vi "FRCts20_Backend_ClosedRequests.vi"(6 "Message Attributes":T1, 8 "error in (no error)":errorcluster, 10 "Data":string, 11 "Engine_Refnums":T2) -> (0 "error out":errorcluster)   [LabVIEW 2013, in "FRCts20_Backend_Engine.lvlib"]
uses:
  FRCts20_Backend_Engine.lvlib
  FRCts20_Backend_EngineRefnums.ctl
  INI_Accessor/FRCts20_Backend_INI Controller.lvclass
  Dependencies/AMC/_SubVIs/TypeDefs/Message Queue.ctl
  Dependencies/AMC/_SubVIs/TypeDefs/Message.ctl
  Dependencies/Keyed Array/KeyedArray.ctl
  <vilib>/addons/database/Connection.llb/Conn ObjectReference.ctl
  FRCts20_Backend_FGVOperation.ctl
  FRCts20_Backend_API/FRCts20_Backend_API_ClosedRequests.ctl
  FRCts20_Backend_API/FRCts20_Backend_API.lvlib
  Dependencies/Keyed Array/Tools_KeyedArray.lvlib
  Dependencies/AMC/AMC.lvlib
  <vilib>/addons/database/NI_Database_API.lvlib
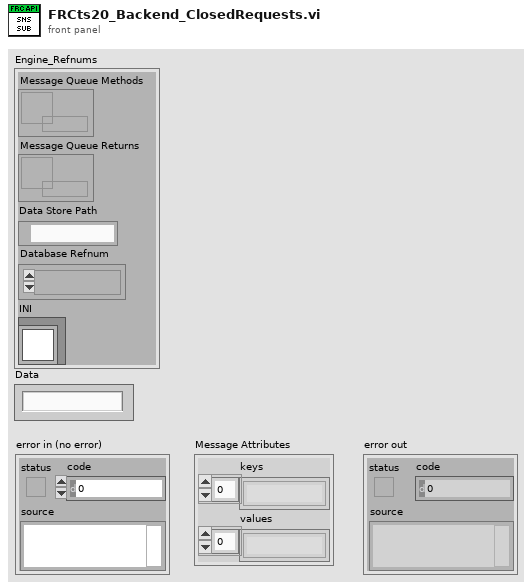
[diagram p1: front panel]
types:
  T1 = typedef "Tools_KeyedArray.lvlib/KeyedArray.ctl" = cluster{"keys":string[], "values":string[]}
  T2 = typedef "FRCts20_Backend_Engine.lvlib/FRCts20_Backend_EngineRefnums.ctl" = cluster{"Message Queue Methods":T3, "Message Queue Returns":T3, "Data Store Path":path, "Database Refnum":T4, "INI":refnum<class "FRCts20_Backend_INI Controller.lvclass">}
  T3 = typedef "AMC.lvlib/Message Queue.ctl" = refnum<queue>
  T4 = typedef "NI_Database_API.lvlib/Conn ObjectReference.ctl" = refnum<k1>
  T5 = typedef "FRCts20_Backend_API.lvlib/FRCts20_Backend_API_ClosedRequests.ctl" = cluster{"Event Name":string, "APIReturn":string, "Array of Requests":cluster{"Team Number":string, "ReqNumber":string, "Request":string, "OpenDate":string, "CloseDate":string}[]}
  T6 = typedef "FRCts20_Backend_Engine.lvlib/FRCts20_Backend_FGVOperation.ctl" = enum16{"Initialize", "EnqueueMessage", "EnqueueDataReturn", "FlushMessage", "FlushDataReturn"}
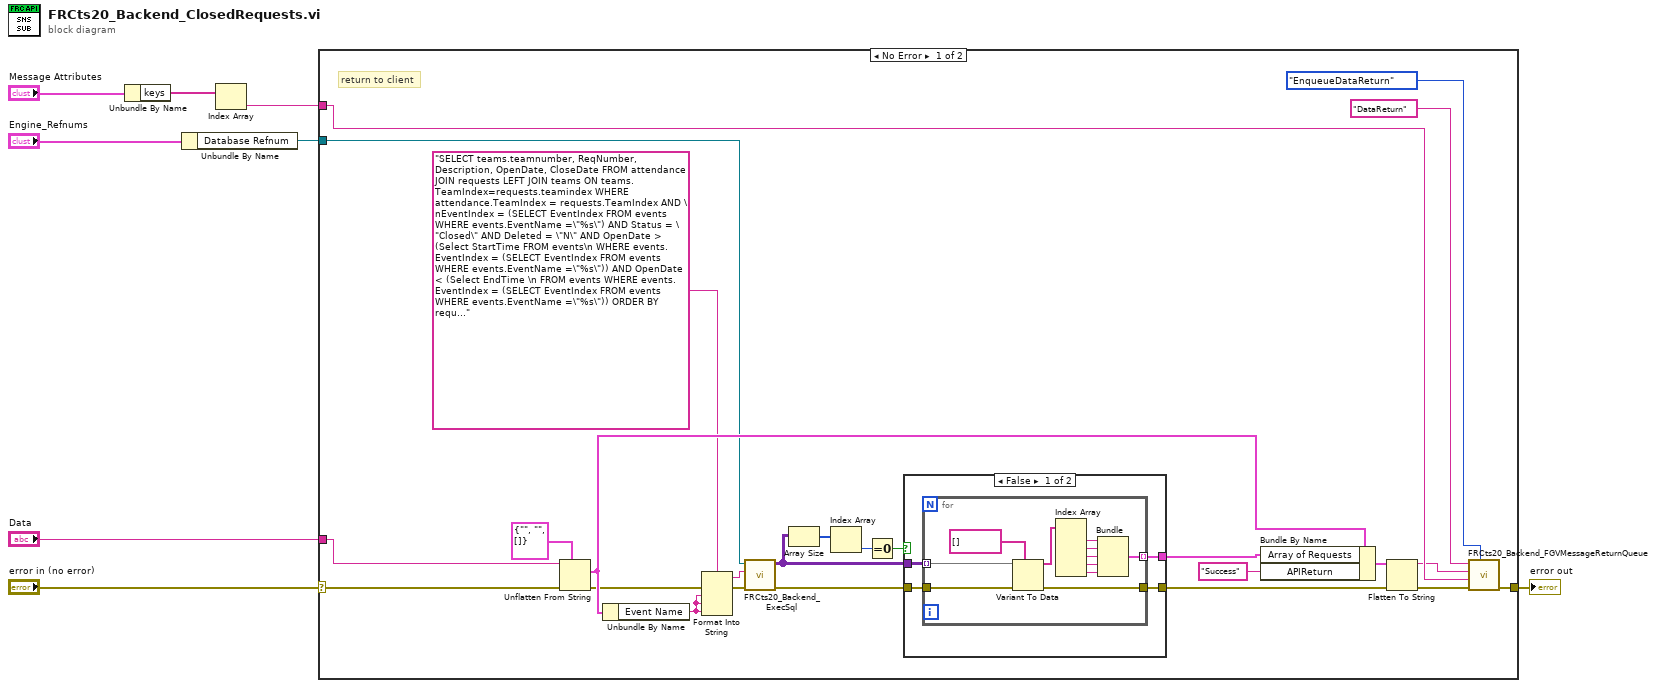
[diagram p0: block diagram]
diagram:
  n1 = Unbundle By Name("Message Attributes") -> ("keys"=w4:string[])
  n2 = Unbundle By Name("Engine_Refnums") -> ("Database Refnum"=w1:T4)
  n3 = Index Array(array=w4) -> (element=w3:string)  [unwired: 1 in]
  n4 = case shown="No Error" "error in (no error)" {
    selector: "error in (no error)" -> [w31 w50]
    tunnel: [w12 w50] -> w7
    tunnel: w1 -> [w19 _]
    tunnel: "Data" -> [w32 _]
    tunnel: w3 -> [w33 _]
    frame No Error {
      # "return to client"
      n5 = Unflatten From String(type=T5 {"Event Name"="", "APIReturn"="", "Array of Requests"=[]} ("ClosedRequests"), binary string=w32, error in (no error)=w31) -> (value=w28:T5, error out=w18:errorcluster)  [unwired: 2 in, 1 out]
      n6 = Unbundle By Name(w28) -> ("Event Name"=w20:string)
      n7 = Format Into String(format string="SELECT teams.teamnumber, ReqNumber, Description, OpenDate, CloseDate FROM attendance JOIN requests LEFT JOIN teams ON teams.TeamIndex=requests.teamindex WHERE attendance.TeamIndex = requests.TeamIndex AND \nEventIndex = (SELECT EventIndex FROM events WHERE events.EventName =\"%s\") AND Status = \"Closed\" AND Deleted = \"N\" AND OpenDate > (Select StartTime FROM events\n WHERE events.EventIndex = (SELECT EventIndex FROM events WHERE events.EventName =\"%s\")) AND OpenDate < (Select EndTime \n FROM events WHERE events.EventIndex = (SELECT EventIndex FROM events WHERE events.EventName =\"%s\")) ORDER BY requests.TeamIndex, ReqNumber", error in=w18, w20, w20, w20) -> (resulting string=w16:string, error out=w17:errorcluster)  [unwired: 1 in]
      n8 = call "FRCts20_Backend_ExecSql.vi"("error in (no error)"=w17, "format string"=w16, "Refnum in"=w19) -> ("error out"=w11:errorcluster, "recordset data"=w15:variant[][])  [unwired: 6 in, 1 out]
      n9 = Array Size(array=w15) -> (size(s)=w23:i32[])
      n10 = Index Array(array=w23) -> (element=w14:i32)  [unwired: 1 in]
      n11 = Equal To 0?(x=w14) -> (x = 0?=w22:bool)
      n12 = case shown="False" w22 {
        tunnel: w15 -> [w37 _]
        tunnel: w11 -> [w36 w49]
        tunnel: [w34 w49] -> w13
        tunnel: [w35 _] -> w9
        frame False {
          n13 = for {
            tunnel: w37 -> [w45] mode=indexing
            tunnel: w36 -> [w44]
            tunnel: [w40] -> w35 mode=indexing
            tunnel: [w38] -> w34
            n14 = Variant To Data(error in=w44, type=string[] [], Variant=w45) -> (data=w43:string[], error out=w38:errorcluster)
            n15 = Index Array(array=w43) -> (element #1=w39:string, element #2=w47:string, element #3=w48:string, element #4=w42:string, element #5=w41:string)  [unwired: 5 in]
            n16 = Bundle(w39, w47, w48, w42, w41) -> (w40:cluster{string, string, string, string, string})  [unwired: 1 in]
          }
        }
        frame True {
        }
      }
      n17 = Bundle By Name(cluster=w28, "Array of Requests"=w9, "APIReturn"="Success") -> (w27:T5)
      n18 = Flatten To String(anything=w27, error in (no error)=w13) -> (data string=w26:string, error out=w25:errorcluster)  [unwired: 2 in, 1 out]
      n19 = call "FRCts20_Backend_FGVMessageReturnQueue.vi"("Operation"=FRCts20_Backend_FGVOperation."EnqueueDataReturn", "error in (no error)"=w25, "Key"=w33, "Message Value"=w26, "Message Name"="DataReturn") -> ("error out"=w12:errorcluster)  [unwired: 5 in, 1 out]
    }
    frame Error {
    }
  }
  "error out" <- w7
